vi "_099.vi"() -> ()   [LabVIEW 2020]
panel:
  out "Array":i32[](array[numeric])
  out "Numeric":i32
  out "Array 2":i32[][](array[numeric])
  out "Array 1":i32[](array[numeric])
  # "What is the data type of Indicator 1 & 2 ?"
  # "Array 1  :\nArray 2 :"
  # "1D Array with integers\n2D Array with integers"
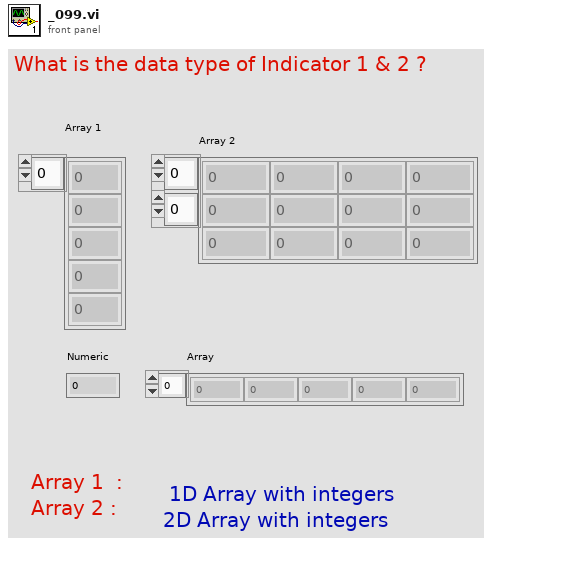
[diagram p1: front panel]
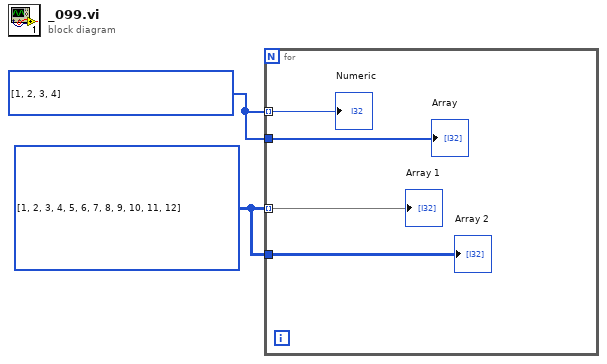
[diagram p0: block diagram]
diagram:
  w1 = i32[] [1, 2, 3, 4]
  w2 = i32[][] [[1, 2, 3, 4], [5, 6, 7, 8], [9, 10, 11, 12]]
  n1 = for {
    tunnel: w2 -> [w6] mode=indexing
    tunnel: w2 -> [w5]
    tunnel: w1 -> [w4] mode=indexing
    tunnel: w1 -> [w3]
    "Array 1" <- w6
    "Array 2" <- w5
    "Numeric" <- w4
    "Array" <- w3
  }
